vi "PV Vent valve controlling turbopump.vi"(8 "error in (no error)":errorcluster, 9 "PV Vent valve controlling - Cluster":T1={"Parameter"=0, "Parameter\nread only<->describe"=FALSE, "Venting enable\n  off     <-------->     on   "=TRUE, "Venting frequency [%]"=50, "Venting time [s]"=3600, "Venting mode"=0} {"Venting mode" items=[" automatic venting", " do not vent", " venting \"ON\""]; "Venting time [s]" min=6 max=3600 step=1; "Venting frequency [%]" min=40 max=80 step=1; "Parameter" items=[" Venting enable [off / on]", " Venting mode  [0=automatic venting; 1=do not vent; 2=venting \"ON\"]", " Venting frequency  as a % of the final rot. speed of the TMP", " Venting time [s]"]}, 10 "Adress of unit":u16=1 min=1 max=999 step=1, 11 "VISA session":refnum<visa-resource-name>) -> (0 "error out":errorcluster, 2 "response (data)":string, 3 "dup VISA session":refnum<visa-resource-name>)   [LabVIEW 2016, in "Pfeiffer Vacuum.lvlib"]
doc: "There are 4 parameters available, only one of which can be enabled at a time. \n\n0 - Venting enable [off / on] (default) (Para.012)\n1 - Venting mode (Para.030)\n [0=automatic venting; 1=do not vent; 2=venting \"ON\"]\n2 - Venting frequency as a % of the final rot. speed of the TMP (Para.720)\n3 - Venting time [s] (Para.721)\n\nNote: The 4 controls right of this one will set the appropriate values for the selected parameter. Any settings for an parameter that is not selected will be ignored. If a value is out of range, it will be changed to either the upper or the lower limit of the range."
uses:
  Pfeiffer Vacuum.lvlib
  PV Ventig time - Cluster.ctl
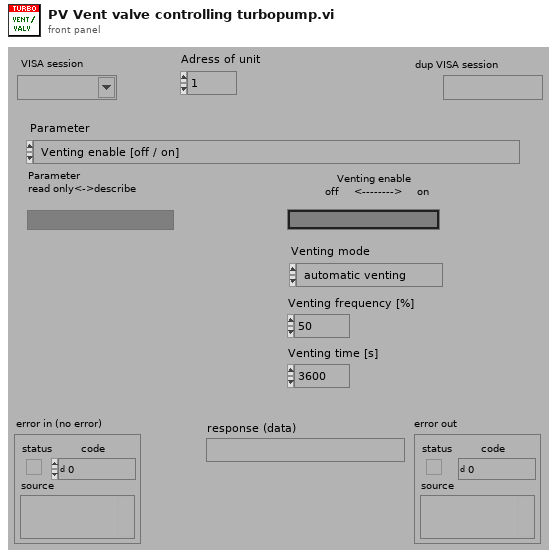
[diagram p1: front panel]
types:
  T1 = typedef "Pfeiffer Vacuum.lvlib/PV Ventig time - Cluster.ctl" = cluster{"Parameter":u16, "Parameter\nread only<->describe":bool, "Venting enable\n  off     <-------->     on   ":bool, "Venting frequency [%]":u16, "Venting time [s]":u16, "Venting mode":u16}
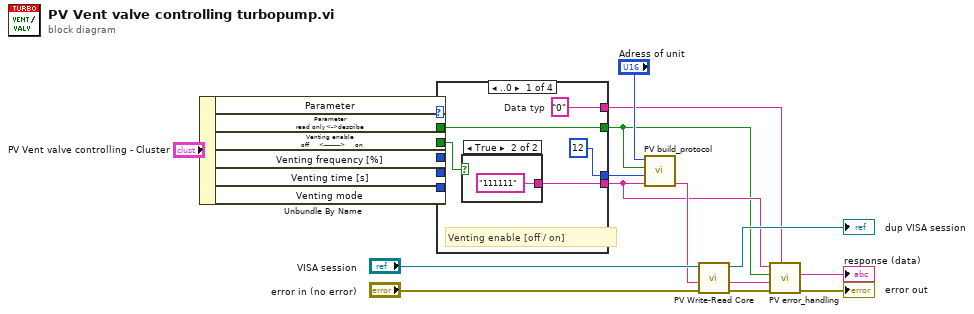
[diagram p0: block diagram]
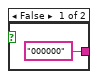
[diagram p2: hidden frame]
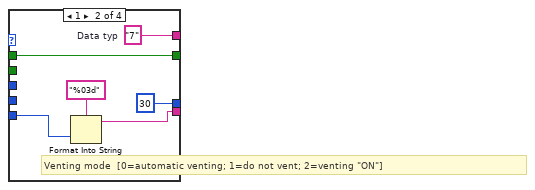
[diagram p3: hidden frame]
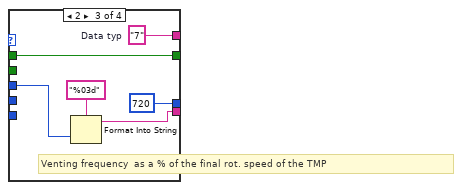
[diagram p4: hidden frame]
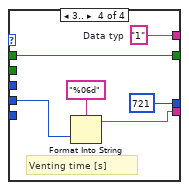
[diagram p5: hidden frame]
diagram:
  n1 = Unbundle By Name("PV Vent valve controlling - Cluster") -> ("Parameter"=w17:u16, "Parameter\nread only<->describe"=w16:bool, "Venting enable\n  off     <-------->     on"=w15:bool, "Venting frequency [%]"=w13:u16, "Venting time [s]"=w12:u16, "Venting mode"=w14:u16)
  n2 = case shown="..0" w17 {
    tunnel: [u16 12 ("Parameter-number") u16 30 ("Parameter-number") u16 720 ("Parameter-number") u16 721 ("Parameter-number")] -> w19
    tunnel: [w24 w31 w37 w43] -> w2
    tunnel: [w23 w32 w38 w44] -> w1
    tunnel: w16 -> [w23 w32 w38 w44]
    tunnel: w15 -> [w22 _ _ _]
    tunnel: w14 -> [_ w29 _ _]
    tunnel: w13 -> [_ _ w35 _]
    tunnel: w12 -> [_ _ _ w41]
    tunnel: [w21 w28 w34 w40] -> w3
    frame ..0 {
      w21 = "0"  # Data typ
      # "Venting enable [off / on]"
      n3 = case shown="True" w22 {
        tunnel: ["000000" ("Data") "111111" ("Data")] -> w24
        frame False {
        }
        frame True {
        }
      }
    }
    frame 1 {
      w28 = "7"  # Data typ
      # "Venting mode  [0=automatic venting; 1=do not vent; 2=venting \"ON\"]"
      n4 = Format Into String(format string="%03d" ("Format-String"), w29) -> (resulting string=w31:string)  [unwired: 2 in, 1 out]
    }
    frame 2 {
      w34 = "7"  # Data typ
      # "Venting frequency  as a % of the final rot. speed of the TMP"
      n5 = Format Into String(format string="%03d" ("Format-String"), w35) -> (resulting string=w37:string)  [unwired: 2 in, 1 out]
    }
    frame 3.. {
      w40 = "1"  # Data typ
      # "Venting time [s]"
      n6 = Format Into String(format string="%06d" ("Format-String"), w41) -> (resulting string=w43:string)  [unwired: 2 in, 1 out]
    }
  }
  n7 = call "PV build_protocol.vi"("Data"=w2, "Parameter-number"=w19, "parameter\nread<->describe"=w1, "Adress"="Adress of unit") -> ("output"=w9:string)  [unwired: 3 in]
  n8 = call "PV Write-Read Core.vi"("error in"="error in (no error)", "Write data in"=w9, "VISA session"="VISA session") -> ("error out"=w6:errorcluster, "response (data) out"=w7:string, "dup VISA session"=→"dup VISA session":refnum<visa-resource-name>)  [unwired: 2 in]
  n9 = call "PV error_handling.vi"("Data Typ in"=w3, "error in"=w6, "response (data) in"=w7, "Parameter\nread only<->describe"=w1, "data in"=w2) -> ("error out"=→"error out":errorcluster, "Data out"=→"response (data)":string)  [unwired: 4 in, 1 out]
